vi "Configure Acquisition Type.vi"(8 "error in (no error)":errorcluster, 9 "Number of segments (10)":i16=10, 10 "Acquisition Type (0: Normal)":u16(ring) items=["Normal", "Sequence"], 11 "VISA resource name":refnum<visa-resource-name>) -> (0 "error out":errorcluster, 3 "VISA resource name out":refnum<visa-resource-name>)   [LabVIEW 2015, in "LeCroy Wave Series.lvlib"]
doc: "Sets the conditions for the sequence mode acquisition.\n\nNote:\nThis VI has been obsoleted from the driver and is included for compatibility with existing applications. New applications should use the Configure Sample Mode."
uses:
  <instrlib>/LeCroy Wave Series/LeCroy Wave Series.lvlib
panel:
  # "Note:\nThis VI has been obsoleted from the driver and is included for compatibility with existing applications.  New applications should use the Configure Sample Mode."
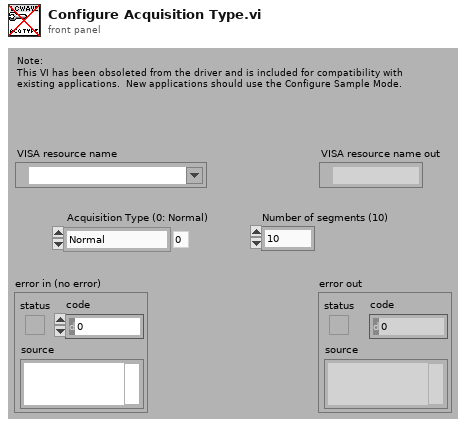
[diagram p1: front panel]
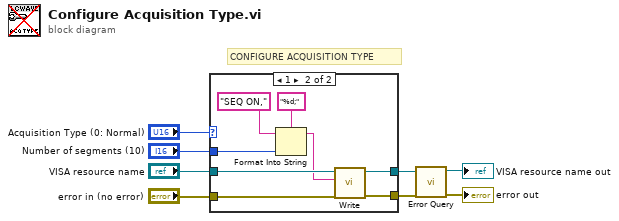
[diagram p0: block diagram]
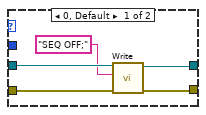
[diagram p2: hidden frame]
diagram:
  # "CONFIGURE ACQUISITION TYPE"
  n1 = case shown="1" "Acquisition Type (0: Normal)" {
    tunnel: "VISA resource name" -> [w11 w21]
    tunnel: "error in (no error)" -> [w10 w20]
    tunnel: [w12 w19] -> w6
    tunnel: [w13 w18] -> w3
    tunnel: "Number of segments (10)" -> [_ w14]
    frame 0, Default {
      n2 = call <instrlib>:"Write.vi"("error in (no error)"=w10, "Write Buffer"="SEQ OFF;", "VISA resource name"=w11) -> ("error out"=w13:errorcluster, "VISA resource name out"=w12:refnum<visa-resource-name>)  [unwired: 6 in, 1 out]
    }
    frame 1 {
      n3 = Format Into String(format string="%d;", initial string="SEQ ON,", w14) -> (resulting string=w15:string)  [unwired: 1 in, 1 out]
      n4 = call <instrlib>:"Write.vi"("error in (no error)"=w20, "Write Buffer"=w15, "VISA resource name"=w21) -> ("error out"=w18:errorcluster, "VISA resource name out"=w19:refnum<visa-resource-name>)  [unwired: 6 in, 1 out]
    }
  }
  n5 = call <instrlib>:"Error Query.vi"("error in (no error)"=w3, "VISA resource name"=w6) -> ("error out"=→"error out":errorcluster, "VISA resource name out"=→"VISA resource name out":refnum<visa-resource-name>)  [unwired: 6 in, 2 out]
